vi "UI.vi"(8 "error in (no error)":errorcluster, 11 "Node Ptr":T1 format="%.0x") -> (0 "error out":errorcluster)   [LabVIEW 2017, in "Modules.lvlib" / "9253.lvclass"]
uses:
  9253.lvclass
  <vilib>/NI Veristand/Custom Device API/Custom Device Item Ref.ctl
  RSI Module/SubPanel Command.ctl
  C:/Users/nitest/Documents/NI/niveristand-scan-engine-module-libraries/Source/RSI Module/RSI Module.lvclass
  9253.lvclass/9253.ctl
  RSI Module/RSI Module.lvclass
  <vilib>/NI Veristand/Custom Device API/Custom Device API.lvlib
panel:
  in  "Butterworth cutoff frequency":u32(ring) items=["4000 Hz", "2000 Hz", "1000 Hz", "500 Hz", "250 Hz", "125 Hz"]
  in  "Filter response":u32(ring) items=["Comb"=0, "Butterworth"=2]
  in  "Butterworth filter order":u32(ring)=1 items=["Order 2"=1, "Order 4"=3]
  in  "Comb frequency":u32(ring) items=["Data rate", "Data rate / 2", "Data rate / 4", "Data rate / 8", "Data rate / 16"]
  in  "Data rate":u32(ring) items=["50.000 kS/s"=0, "33.333 kS/s"=1, "25.000 kS/s"=2, "20.000 kS/s"=3, "16.667 kS/s"=4, "14.286 kS/s"=5, "12.500 kS/s"=6, "11.111 kS/s"=7, "10.000 kS/s"=8, "8.333 kS/s"=9, "7.143 kS/s"=10, "6.250 kS/s"=11, "5.556 kS/s"=12, "5.000 kS/s"=13, "4.545 kS/s"=14, "4.167 kS/s"=15, "3.571 kS/s"=16, "3.125 kS/s"=17, "2.778 kS/s"=18, "2.500 kS/s"=19, "2.273 kS/s"=20, "2.083 kS/s"=21, "2.000 kS/s"=22, "1.786 kS/s"=23, "1.563 kS/s"=24, "1.389 kS/s"=25, "1.250 kS/s"=26, "1.136 kS/s"=27, "1.042 kS/s"=28, "1.000 kS/s"=29, "892.86 S/s"=30, "781.25 S/s"=31, "694.44 S/s"=32, "625.00 S/s"=33, "568.18 S/s"=34, "520.83 S/s"=35, "500.00 S/s"=36, "446.43 S/s"=37, "400.00 S/s"=38, "390.63 S/s"=39, "347.22 S/s"=40, "312.50 S/s"=41, "284.09 S/s"=42, "260.42 S/s"=43, "250.00 S/s"=44, "223.21 S/s"=45, "200.00 S/s"=46, "195.31 S/s"=47, "142.05 S/s"=48, "125.00 S/s"=49, "100.00 S/s"=50, "97.66 S/s"=51, "60.02 S/s"=52, "50.00 S/s"=54, "10.00 S/s"=56]
  in  "_Update Chan Settings":bool
  in  "SubPanel Event":refnum<user-event>
  in  "Header":cluster{"Section Name":string}={"Section Name"="NI 9253 Settings"}
  # "Each 9253 module supports field-side power fault detection and channel overcurrent detection.\nThese features are not supported by this custom device."
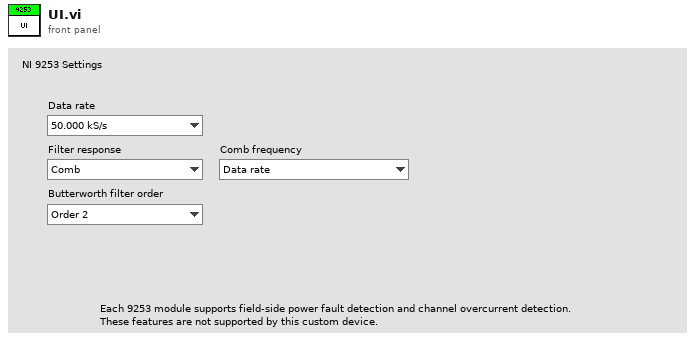
[diagram p1: front panel]
types:
  T1 = typedef "Custom Device API.lvlib/Custom Device Item Ref.ctl" = u64
  T2 = typedef "Modules.lvlib/RSI Module.lvclass/Module Models.ctl" = enum16{"Empty", "NI 9201", "NI 9203", "NI 9205", "NI 9206", "NI 9207", "NI 9208", "NI 9209", "NI 9210", "NI 9211", "NI 9212", "NI 9213", "NI 9214", "NI 9215", "NI 9216", "NI 9217", "NI 9219", "NI 9220", "NI 9221", "NI 9222", "NI 9223", "NI 9224", "NI 9225", "NI 9226", "NI 9227", "NI 9228", "NI 9229", "NI 9233", "NI 9234", "NI 9235", "NI 9236", "NI 9237", "NI 9239", "NI 9242", "NI 9244", "NI 9253", "NI 9263", "NI 9264", "NI 9265", "NI 9266", "NI 9269", "NI 9344", "NI 9350", "NI 9375", "NI 9401", "NI 9402", "NI 9403", "NI 9411", "NI 9421", "NI 9422", "NI 9423", "NI 9425", "NI 9426", "NI 9435", "NI 9436", "NI 9437", "NI 9472", "NI 9474", "NI 9475", "NI 9476", "NI 9477", "NI 9478", "NI 9481", "NI 9482", "NI 9485"}
  T3 = typedef "Modules.lvlib/RSI Module.lvclass/SubPanel Command.ctl" = enum16{"Stop"}
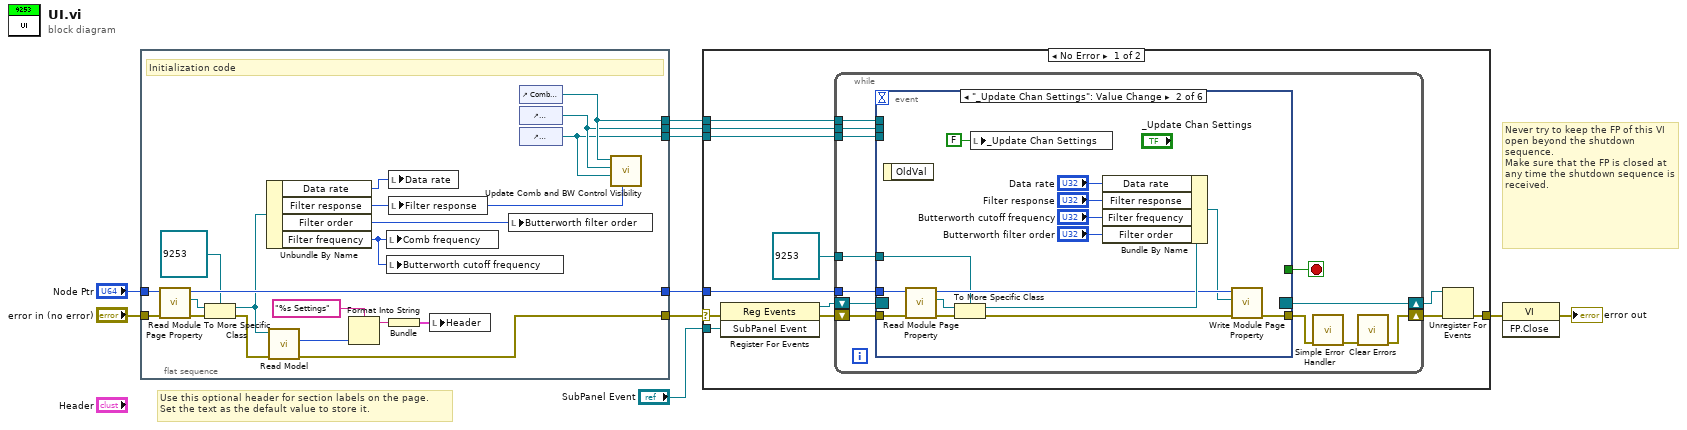
[diagram p0: block diagram]
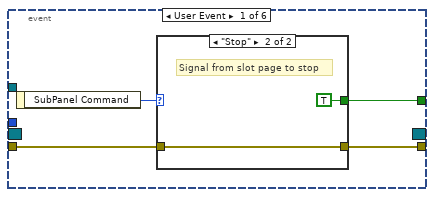
[diagram p2: hidden frame]
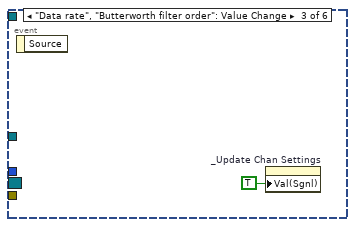
[diagram p4: hidden frame]
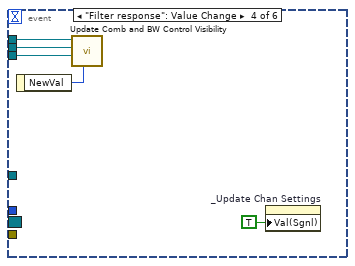
[diagram p5: hidden frame]
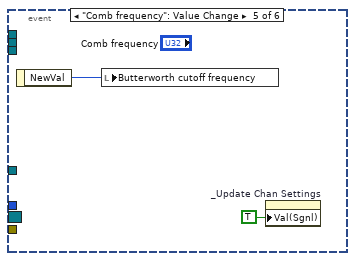
[diagram p6: hidden frame]
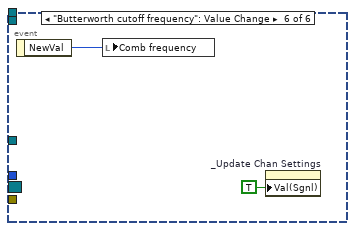
[diagram p7: hidden frame]
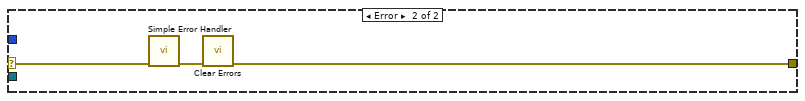
[diagram p8: hidden frame]
diagram:
  # "Never try to keep the FP of this VI open beyond the shutdown sequence.\nMake sure that the FP is closed at any time the shutdown sequence is received."
  # "Use this optional header for section labels on the page. \nSet the text as the default value to store it."
  n1 = flat-sequence {
    tunnel: "error in (no error)" -> [w29]
    tunnel: "Node Ptr" -> [w30]
    tunnel: [w11] -> w4
    tunnel: [w28] -> w7
    tunnel: [w15] -> w3
    tunnel: [w14] -> w2
    tunnel: [w13] -> w1
    frame #0 {
      # "Initialization code"
      n2 = call "Read Module Page Property.vi"("error in (no error)"=w29, "Node Ptr In"=w30) -> ("error out"=w27:errorcluster, "RSI Module"=w25:refnum<class "RSI Module.lvclass">, "Node Ptr Out"=w28:T1)  [unwired: 7 in]
      n3 = To More Specific Class(target class=refnum<class "9253.lvclass"> refnum ("9205 in"), reference=w25, error in=w27) -> (specific class reference=w24:refnum<class "9253.lvclass">, error out=w23:errorcluster)
      n4 = Unbundle By Name(w24) -> ("Data rate"=w18:u32, "Filter response"=w16:u32, "Filter order"=w17:u32, "Filter frequency"=w12:u32)
      n5 = call "Read Model.vi"("error in (no error)"=w23, "RSI Module in"=w24) -> ("error out"=w11:errorcluster, "Model"=w21:T2)  [unwired: 7 in, 1 out]
      n6 = Format Into String(format string="%s Settings", w21) -> (resulting string=w19:string)  [unwired: 2 in, 1 out]
      n7 = local write "Comb frequency"(w12) -> ()
      n8 = local write "Butterworth cutoff frequency"(w12) -> ()
      n9 = local write "Data rate"(w18) -> ()
      n10 = local write "Filter response"(w16) -> ()
      n11 = Bundle(w19) -> (w22:cluster{string})  [unwired: 1 in]
      n12 = local write "Header"(w22) -> ()
      n13 = local write "Butterworth filter order"(w17) -> ()
      n14 = control-ref of="Comb frequency"() -> (w15:refnum<vi>)
      n15 = control-ref of="Butterworth filter order"() -> (w14:refnum<vi>)
      n16 = control-ref of="Butterworth cutoff frequency"() -> (w13:refnum<vi>)
      n17 = call "Update Comb and BW Control Visibility.vi"("Filter response"=w16, "Butterworth filter order"=w13, "Butterworth cutoff frequency"=w14, "comb frequency"=w15) -> ()  [unwired: 6 in]
    }
  }
  n18 = case shown="No Error" w4 {
    selector: w4 -> [w36 w89]
    tunnel: [w40 w87] -> w10
    tunnel: w7 -> [w37 _]
    tunnel: "SubPanel Event" -> [w35 _]
    tunnel: w3 -> [w34 _]
    tunnel: w2 -> [w33 _]
    tunnel: w1 -> [w32 _]
    frame No Error {
      n19 = register-events(error in=w36, w35) -> (reference out=w38:refnum<event-registration>, error out=w39:errorcluster)  [unwired: 1 in]
      n20 = while {
        tunnel: w37 -> [w50]
        shift-right: [w47] -> w41
        shift-left: w39 -> [w53]
        shift-right: [w54] -> w42
        shift-left: w38 -> [w52]
        tunnel: w34 -> [w46]
        tunnel: w33 -> [w45]
        tunnel: w32 -> [w44]
        tunnel: refnum<class "9253.lvclass"> refnum ("9205 in") -> [w43]
        stop <- w51 stop-if-true
        n21 = event shown="[1] \"_Update Chan Settings\": Value Change" {
          selector: w52 -> [_ _ _ _ _ _]
          dyn-events: [_ _ _ _ _ _] -> w54
          timeout: _ -> [_ _ _ _ _ _]
          tunnel: w53 -> [w57 w69 _ _ _ _]
          tunnel: [w56 _ _ _ _ _] -> w51
          tunnel: [w55 w68 _ _ _ _] -> w49
          tunnel: w50 -> [_ w70 _ _ _ _]
          tunnel: w46 -> [_ _ _ w80 _ _]
          tunnel: w45 -> [_ _ _ w79 _ _]
          tunnel: w44 -> [_ _ _ w78 _ _]
          tunnel: w43 -> [_ w67 _ _ _ _]
          event User Event {
            n22 = event-data() -> ("SubPanel Command"=w58:T3)  [unwired: 1 out]
            n23 = case shown="\"Stop\"" w58 {
              tunnel: w57 -> [w59 w60]
              tunnel: [w59 w60] -> w55
              tunnel: [_ TRUE] -> w56
              frame Default {
              }
              frame "Stop" {
                # "Signal from slot page to stop"
              }
            }
          }
          event "_Update Chan Settings": Value Change {
            n24 = event-data() -> ()  [unwired: 2 out]
            n25 = call "Read Module Page Property.vi"("error in (no error)"=w69, "Node Ptr In"=w70) -> ("error out"=w75:errorcluster, "RSI Module"=w76:refnum<class "RSI Module.lvclass">, "Node Ptr Out"=w72:T1)  [unwired: 7 in]
            n26 = To More Specific Class(target class=w67, reference=w76, error in=w75) -> (specific class reference=w74:refnum<class "9253.lvclass">, error out=w73:errorcluster)
            n27 = local write "_Update Chan Settings"(FALSE ("_Update Values")) -> ()
            n28 = Bundle By Name(cluster=w74, "Data rate"="Data rate", "Filter response"="Filter response", "Filter frequency"="Butterworth cutoff frequency", "Filter order"="Butterworth filter order") -> (w71:refnum<class "9253.lvclass">)
            n29 = call "Write Module Page Property.vi"("error in (no error)"=w73, "RSI Module"=w71, "Node Ptr In"=w72) -> ("error out"=w68:errorcluster)  [unwired: 6 in, 2 out]
          }
          event "Data rate", "Butterworth filter order": Value Change {
            n30 = event-data() -> ()  [unwired: 2 out]
            n31 = property on="_Update Chan Settings" class="Bool (strict)"("Val(Sgnl)"=TRUE ("Value (Signaling)")) -> ()  [unwired: 2 in, 2 out]
          }
          event "Filter response": Value Change {
            n32 = event-data() -> ("NewVal"=w81:u32)  [unwired: 1 out]
            n33 = call "Update Comb and BW Control Visibility.vi"("Filter response"=w81, "Butterworth filter order"=w78, "Butterworth cutoff frequency"=w79, "comb frequency"=w80) -> ()  [unwired: 6 in]
            n34 = property on="_Update Chan Settings" class="Bool (strict)"("Val(Sgnl)"=TRUE ("Value (Signaling)")) -> ()  [unwired: 2 in, 2 out]
          }
          event "Comb frequency": Value Change {
            n35 = event-data() -> ("NewVal"=w83:u32)  [unwired: 1 out]
            n36 = local write "Butterworth cutoff frequency"(w83) -> ()
            n37 = property on="_Update Chan Settings" class="Bool (strict)"("Val(Sgnl)"=TRUE ("Value (Signaling)")) -> ()  [unwired: 2 in, 2 out]
          }
          event "Butterworth cutoff frequency": Value Change {
            n38 = event-data() -> ("NewVal"=w85:u32)  [unwired: 1 out]
            n39 = local write "Comb frequency"(w85) -> ()
            n40 = property on="_Update Chan Settings" class="Bool (strict)"("Val(Sgnl)"=TRUE ("Value (Signaling)")) -> ()  [unwired: 2 in, 2 out]
          }
        }
        n41 = call <vilib>:"Simple Error Handler.vi"("error in (no error)"=w49) -> ("error out"=w48:errorcluster)  [unwired: 1 in, 7 out]
        n42 = call <vilib>:"Clear Errors.vi"("error in (no error)"=w48) -> ("error out"=w47:errorcluster)  [unwired: 1 in, 5 out]
      }
      n43 = Unregister For Events(event registration refnum=w42, error in=w41) -> (error out=w40:errorcluster)
    }
    frame Error {
      n44 = call <vilib>:"Simple Error Handler.vi"("error in (no error)"=w89) -> ("error out"=w88:errorcluster)  [unwired: 1 in, 7 out]
      n45 = call <vilib>:"Clear Errors.vi"("error in (no error)"=w88) -> ("error out"=w87:errorcluster)  [unwired: 1 in, 5 out]
    }
  }
  n46 = invoke class="VI" method="FP.Close"(error in=w10) -> (error out=→"error out":errorcluster)  [unwired: 2 in, 2 out]
